vi "AttrGet.vi"   [LabVIEW 2011, in "Konvolucio MUDS150628.lvlib"]
uses:
  <instrlib>/Konvolucio MUDS150628/Konvolucio MUDS150628.lvlib
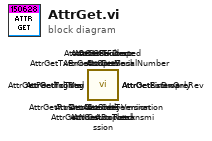
[diagram p0: block diagram]
diagram:
  n1 = call <instrlib>:"AttrGetAssemblyVersion.vi"() -> ()  [unwired: 9 in, 3 out]
  n2 = call <instrlib>:"AttrGetSerialNumber.vi"() -> ()  [unwired: 9 in, 3 out]
  n3 = call <instrlib>:"AttrGetPcbRev.vi"() -> ()  [unwired: 9 in, 3 out]
  n4 = call <instrlib>:"AttrGetFirmwareRev.vi"() -> ()  [unwired: 9 in, 3 out]
  n5 = call <instrlib>:"AttrGetNonAutoRetransmission.vi"() -> ()  [unwired: 9 in, 3 out]
  n6 = call <instrlib>:"AttrGetIsConnected.vi"() -> ()  [unwired: 9 in, 3 out]
  n7 = call <instrlib>:"AttrGetIsOpen.vi"() -> ()  [unwired: 9 in, 3 out]
  n8 = call <instrlib>:"AttrGetPendingMsg.vi"() -> ()  [unwired: 9 in, 3 out]
  n9 = call <instrlib>:"AttrGetTermination.vi"() -> ()  [unwired: 9 in, 3 out]
  n10 = call <instrlib>:"AttrGetListenOnly.vi"() -> ()  [unwired: 9 in, 3 out]
  n11 = call <instrlib>:"AttrGetLoopback.vi"() -> ()  [unwired: 9 in, 3 out]
  n12 = call <instrlib>:"AttrGetFilter.vi"() -> ()  [unwired: 9 in, 3 out]
  n13 = call <instrlib>:"AttrGetMask.vi"() -> ()  [unwired: 9 in, 3 out]
  n14 = call <instrlib>:"AttrGetState.vi"() -> ()  [unwired: 9 in, 3 out]
  n15 = call <instrlib>:"AttrGetTxDrop.vi"() -> ()  [unwired: 9 in, 3 out]
  n16 = call <instrlib>:"AttrGetTxTotal.vi"() -> ()  [unwired: 9 in, 3 out]
  n17 = call <instrlib>:"AttrGetTxErrorCounter.vi"() -> ()  [unwired: 9 in, 3 out]
  n18 = call <instrlib>:"AttrGetRxDrop.vi"() -> ()  [unwired: 9 in, 3 out]
  n19 = call <instrlib>:"AttrGetRxTotal.vi"() -> ()  [unwired: 9 in, 3 out]
  n20 = call <instrlib>:"AttrGetRxErrorCounter.vi"() -> ()  [unwired: 9 in, 3 out]
  n21 = call <instrlib>:"AttrGetBaudrate.vi"() -> ()  [unwired: 9 in, 3 out]
